vi "O_Curve_in_Excel.vi"() -> ()   [LabVIEW 2020]
uses:
  <vilib>/addons/_office/NI_ReportGenerationToolkit.lvlib
  <vilib>/Utility/NIReport.llb/Excel/NI_Excel.lvclass
  <vilib>/Utility/NIReport.llb/NI_report.lvclass
  <vilib>/Utility/NIReport.llb/Report Type.ctl
  <vilib>/Utility/NIReport.llb/NI_ReportGenerationCore.lvlib
  <vilib>/addons/_office/excel.llb/Excel Easy Table (num).vi
panel:
  in  "DUMMY":dbl[][](array[numeric])=[[1.0], [2.0], [3.0], [4.0], [5.0], [6.0], [7.0], [8.0], [9.0], [10.0], [11.0], [12.0], [13.0], [14.0], [15.0], [16.0], [17.0], [18.0], [19.0], [20.0]] format="%_9g"
  in  "Diff Condition per DUT":dbl
  in  "error in (no error)":errorcluster
  out "error out":errorcluster
  in  "REQUEST #":string
  in  "PROJECT #":string
  # "Column 2"
  # "Column 3"
  # "Column 4"
  # "Column 5"
  # "Column 6"
  # "Column 7"
  # "Column 8"
  # "Column 9"
  # "Column 10"
  # "Column 11"
  # "Column 12"
  # "Column 13"
  # "Column 14"
  # "Column 15"
  # "Column 16"
  # "Column 17"
  # "Column 18"
  # "Column 19"
  # "Column 20"
  # "Column 21"
  # "Column 22"
  # "Column 23"
  # "Column 24"
  # "Column 0"
  # "Column 1"
  # "----------------Already Calculated---------------------"
  # "Tdon\n(ns)"
  # "Tr\n(ns)"
  # "Tdoff\n(ns)"
  # "Tf\n(ns)"
  # "on\ndi (A)"
  # "on\ndt (ns)"
  # "off\ndi (A)"
  # "off\ndt (ns)"
  # "on\ndv (V)"
  # "on\ndt (ns)"
  # "off\ndv (V)"
  # "off\ndt (ns)"
  # "Eon\n(uj)"
  # "Eoff\n(uj)"
  # "di/dt (on)\nA/us"
  # "di/dt (off)\nA/us"
  # "dv/dt (on)\nV/us"
  # "dv/dt (off)\nV/us"
  # "NULL\n(Separator)"
  # "Vce"
  # "Ice"
  # "Vge"
  # "Rg"
  # "Temperature"
  # "DUT  #"
  # "TEST #"
  # "Observation :\n\nTest# 1 - 10 = Diff RG\nTest#11 - 20 = Diff IC"
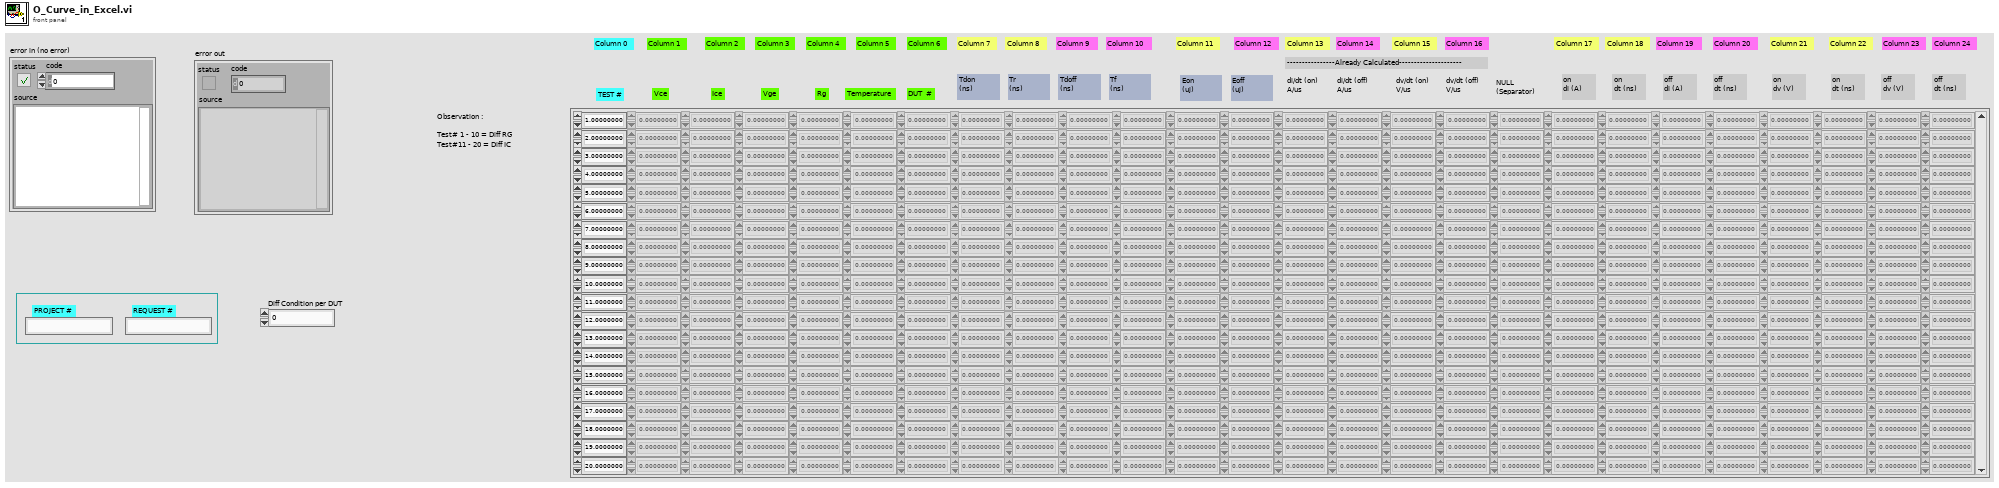
[diagram p1: front panel]
types:
  T1 = typedef "NI_ReportGenerationCore.lvlib/Report Type.ctl" = enum16{"HTML", "Word", "Excel"}
  T2 = enum16{"maximized", "minimized", "normal", "no change"}
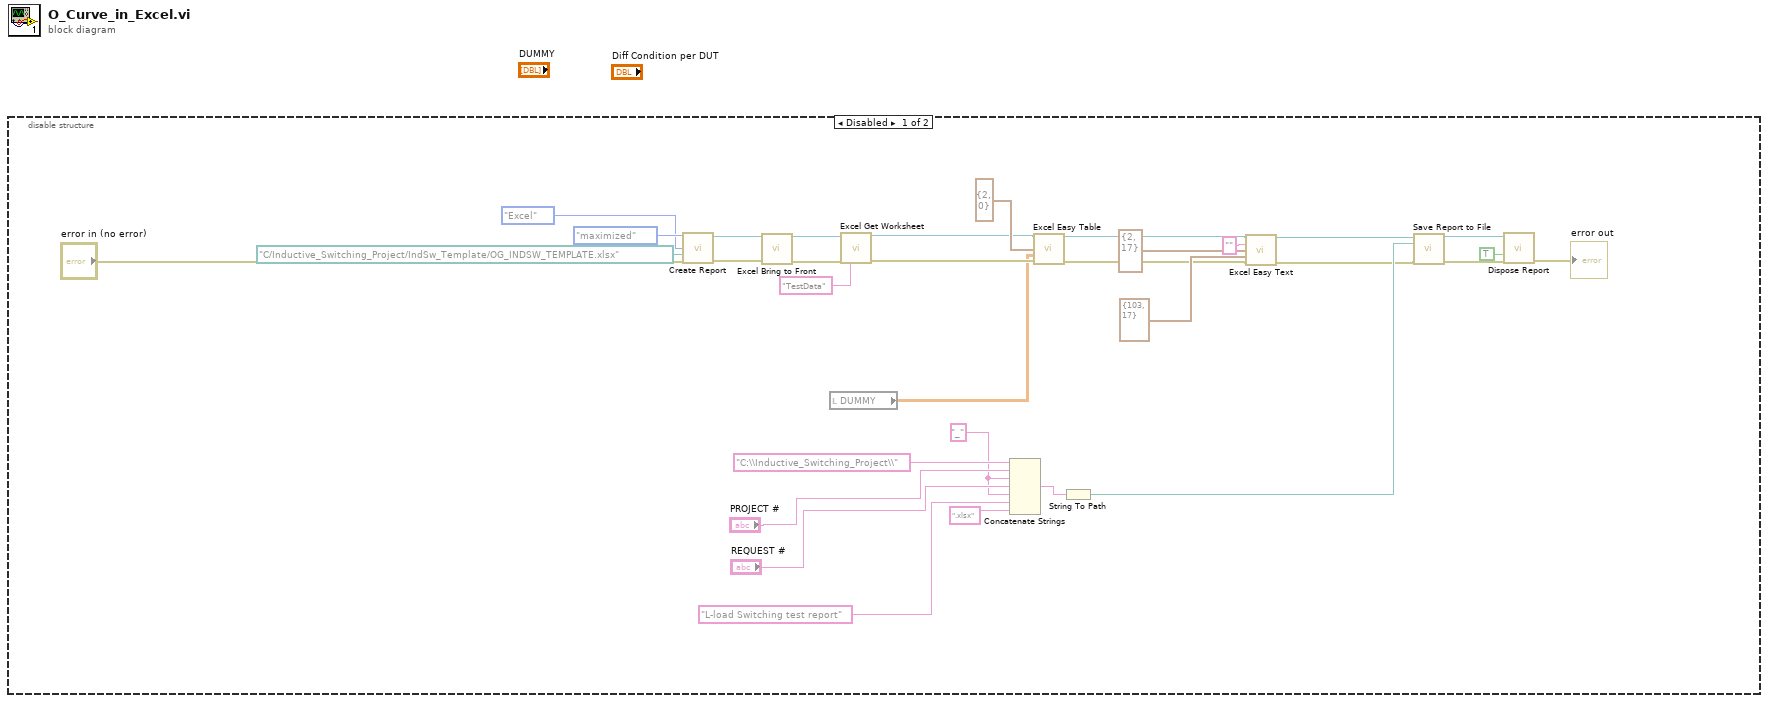
[diagram p0: block diagram]
diagram:
  n1 = disable-structure shown="Disabled" {
    frame Disabled {
      w14 = "_" ("string")
      n2 = call <vilib>:"Create Report.vi"("window state (normal)"=T2."maximized", "report type"=Report_Type."Excel", "template (empty)"=path "C:/Inductive_Switching_Project/IndSw_Template/OG_INDSW_TEMPLATE.xlsx", "error in (no error)"="error in (no error)") -> ("report out"=w10:refnum<class "NI_report.lvclass">, "error out"=w12:errorcluster)  [unwired: 10 in]
      n3 = call <vilib>:"Excel Bring to Front.vi"("report in"=w10, "error in (no error)"=w12) -> ("report out"=w9:refnum<class "NI_report.lvclass">, "error out"=w11:errorcluster)  [unwired: 12 in]
      n4 = local read "DUMMY"() -> (w1:dbl[][])
      n5 = call <vilib>:"Excel Get Worksheet.vi"("report in"=w9, "error in (no error)"=w11, "name (\"\")"="TestData" ("name (\"\")")) -> ("report out"=w22:refnum<class "NI_report.lvclass">, "error out"=w23:errorcluster)  [unwired: 11 in]
      n6 = Concatenate Strings("C:\\Inductive_Switching_Project\\" ("string"), "PROJECT #", w14, "REQUEST #", w14, "L-load Switching test report" ("string"), ".xlsx" ("string")) -> (w32:string)
      n7 = call-poly <vilib>:"Excel Easy Table.vi"("report in"=w22, "start (0, 0)"=cluster{"row":i32, "column":i32} {"row"=2, "column"=0}, "text data"=w1, "error in (no error)"=w23) -> ("report out"=w3:refnum<class "NI_report.lvclass">, "error out"=w5:errorcluster)  [unwired: 7 in, 3 out]
      n8 = String To Path(string=w32) -> (path=w21:path)
      n9 = call <vilib>:"Excel Easy Text.vi"("report in"=w3, "text"="", "start (-1, -1)"=cluster{"row":i32, "column":i32} {"row"=2, "column"=17}, "end (-1, -1)"=cluster{"row":i32, "column":i32} {"row"=103, "column"=17}, "error in (no error)"=w5) -> ("report out"=w2:refnum<class "NI_report.lvclass">, "error out"=w4:errorcluster)  [unwired: 6 in, 3 out]
      n10 = call-dynamic "Save Report to File.vi"("report in"=w2, "report file path"=w21, "error in (no error)"=w4) -> ("report out"=w19:refnum<class "NI_report.lvclass">, "error out"=w20:errorcluster)  [unwired: 11 in]
      n11 = call-dynamic "Dispose Report.vi"("report in"=w19, "save changes? (F)"=TRUE, "error in (no error)"=w20) -> ("error out"=→"error out":errorcluster)  [unwired: 12 in]
    }
    frame Enabled {
    }
  }
